vi "Node information GFV.vi"(0 "Index":u8, 1 "Action(GET)":enum16{"GET", "SET"}(ring), 7 "Control in":T1={"STAT user size"=[0, 0, 6, 0, 0, 0, 0, 0, 0, 0, 0, 0, 0, 0, 0, 0], "HW ID"=1, "FW ID"=16, "SID"=16, "LEIN implementation level"=enum."Full implmentation", "Name"=""}, 11 "error in (no error)":errorcluster) -> (8 "Control out":T1={"STAT user size"=[0, 0, 6, 0, 0, 0, 0, 0, 0, 0, 0, 0, 0, 0, 0, 0], "HW ID"=1, "FW ID"=16, "SID"=16, "LEIN implementation level"=enum."Full implmentation", "Name"=""}, 15 "error out":errorcluster)   [LabVIEW 2010]
uses:
  Defenitions/Node properties.ctl
  Defenitions/LEIN implementation levels.ctl
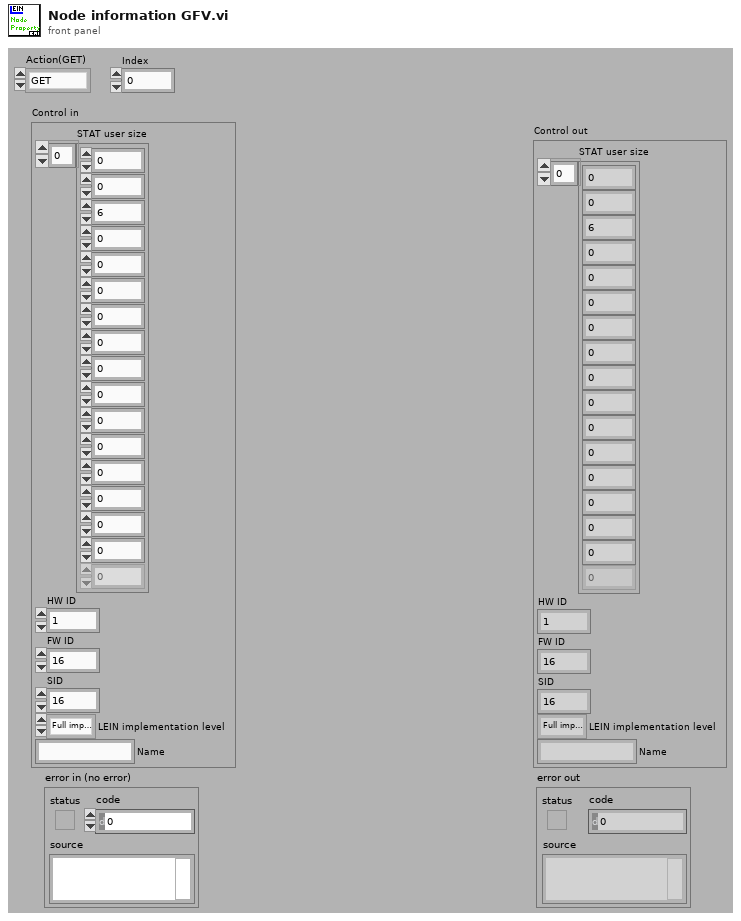
[diagram p1: front panel]
types:
  T1 = typedef "Node properties.ctl" = cluster{"STAT user size":u16[], "HW ID":u8, "FW ID":u8, "SID":u8, "LEIN implementation level":T2, "Name":string}
  T2 = typedef "LEIN implementation levels.ctl" = enum8{"Full implmentation", "Only Stat 2.0"}
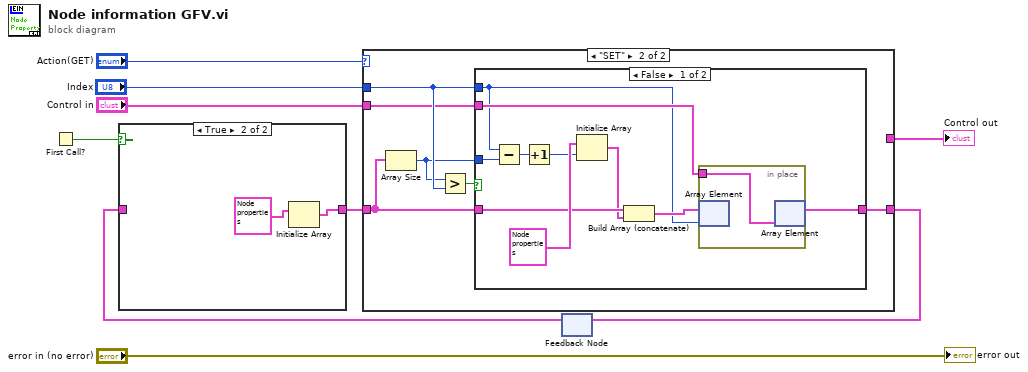
[diagram p0: block diagram]
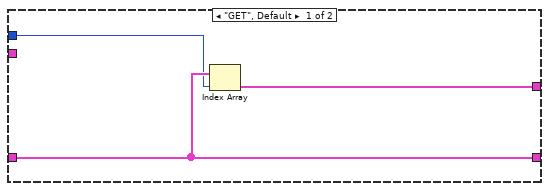
[diagram p3: hidden frame]
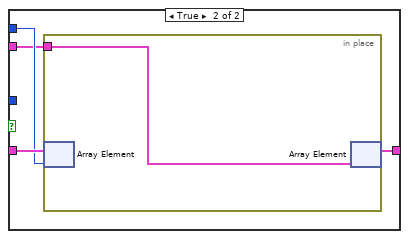
[diagram p4: hidden frame]
diagram:
  n1 = First Call?() -> (First Call?: T/F=w6:bool)
  n2 = feedback #1() -> (w7:T1[])  [unwired: 1 in]
  n3 = case shown="True" w6 {
    tunnel: w7 -> [w10 _]
    tunnel: [w10 w11] -> w4
    frame False {
    }
    frame True {
      n4 = Initialize Array(T1 {"STAT user size"=[0, 0, 0, 0, 0, 0, 0, 0, 0, 0, 0, 0, 0, 0, 0, 0], "HW ID"=1, "FW ID"=16, "SID"=16, "LEIN implementation level"=enum."Full implmentation", "Name"=""} ("Control")) -> (w11:T1[])  [unwired: 1 in]
    }
  }
  n5 = case shown="\"SET\"" "Action(GET)" {
    tunnel: [w15 w21] -> w5
    tunnel: w4 -> [w15 w20]
    tunnel: "Control in" -> [_ w17]
    tunnel: "Index" -> [w14 w18]
    tunnel: [w13 _] -> w1
    frame "GET", Default {
      n6 = Index Array(array=w15, index=w14) -> (element=w13:T1)
    }
    frame "SET" {
      n7 = Array Size(array=w20) -> (size(s)=w16:i32)
      n8 = Greater?(x=w16, y=w18) -> (0:w19:bool)
      n9 = case shown="False" w19 {
        tunnel: [w24 w33] -> w21
        tunnel: w20 -> [w27 w36]
        tunnel: w18 -> [w22 w35]
        tunnel: w17 -> [w23 w34]
        tunnel: w16 -> [w31 _]
        frame False {
          n10 = Subtract(x=w22, y=w31) -> (x-y=w30:i32)
          n11 = Increment(x=w30) -> (x+1=w28:i32)
          n12 = Initialize Array(T1 {"STAT user size"=[0, 0, 0, 0, 0, 0, 0, 0, 0, 0, 0, 0, 0, 0, 0, 0], "HW ID"=1, "FW ID"=16, "SID"=16, "LEIN implementation level"=enum."Full implmentation", "Name"=""} ("Control"), w28) -> (w26:T1[])
          n13 = Build Array (concatenate)(w27, w26) -> (w25:T1[])
          n14 = in-place {
            in-place-border: w23 -> [w32]
            n15 = in-place-array #2(w25, w22) -> ()  [unwired: 1 out]
            n16 = in-place-array #2(w32) -> (w24:T1[])  [unwired: 1 out]
          }
        }
        frame True {
          n17 = in-place {
            in-place-border: w34 -> [w37]
            n18 = in-place-array #3(w36, w35) -> ()  [unwired: 1 out]
            n19 = in-place-array #3(w37) -> (w33:T1[])  [unwired: 1 out]
          }
        }
      }
    }
  }
  "Control out" <- w1
  n20 = feedback-in #1(w5) -> ()
  "error out" <- "error in (no error)"
